vi "Find Cell.vi"(8 "error in":errorcluster, 9 "Lexical Index":string, 10 "Row":refnum<k24>) -> (0 "error out":errorcluster, 2 "Cell":refnum<k24>)   [LabVIEW 2021, in "Open Xml.lvlib"]
uses:
  Open Xml.lvlib
  D:/git/Open-Xml-LabVIEW/Source/DocumentFormat.OpenXml.dll
  DocumentFormat.OpenXml.dll
  D:/git/Open-Xml-LabVIEW/Source/DocumentFormat.OpenXml.Framework.dll
  DocumentFormat.OpenXml.Framework.dll
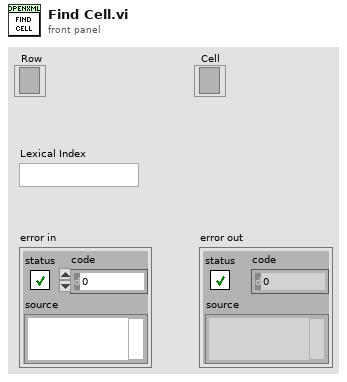
[diagram p1: front panel]
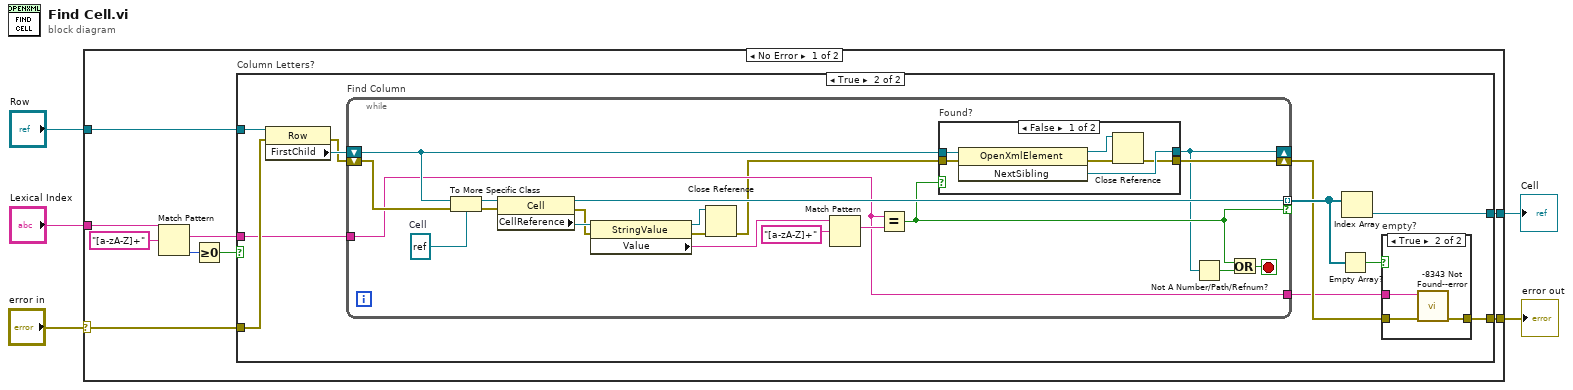
[diagram p0: block diagram]
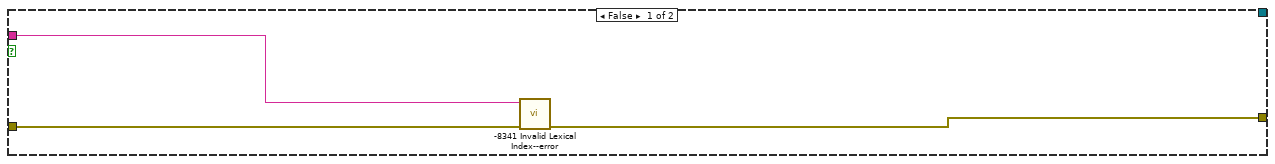
[diagram p2: hidden frame]
diagram:
  n1 = case shown="No Error" "error in" {
    selector: "error in" -> [w13 w61]
    tunnel: "Row" -> [w14 _]
    tunnel: "Lexical Index" -> [w11 _]
    tunnel: [w8 w61] -> w2
    tunnel: [w7 _] -> w1
    frame No Error {
      n2 = Match Pattern(string=w11, regular expression="[a-zA-Z]+") -> (match substring=w10:string, offset past match=w9:i32)  [unwired: 1 in, 2 out]
      n3 = Greater Or Equal To 0?(x=w9) -> (x >= 0?=w6:bool)
      n4 = case "Column Letters?" shown="True" w6 {
        tunnel: w14 -> [_ w28]
        tunnel: w13 -> [w17 w27]
        tunnel: w10 -> [w15 w24]
        tunnel: [w16 w18] -> w8
        tunnel: [_ w23] -> w7
        frame False {
          n5 = call "-8341 Invalid Lexical Index--error.vi"("error in"=w17, "Lexical Index"=w15) -> ("error out"=w16:errorcluster)  [unwired: 9 in]
        }
        frame True {
          n6 = property class="Row"(reference=w28, error in=w27) -> (error out=w25:errorcluster, "FirstChild"=w26:refnum<k24>)  [unwired: 1 out]
          n7 = while "Find Column" {
            shift-right: [w46] -> w20
            shift-left: w25 -> [w52]
            shift-right: [w37] -> _
            shift-left: w26 -> [w36]
            tunnel: [w48] -> w22 mode=indexing if=w38
            tunnel: w24 -> [w35]
            tunnel: [w35] -> w19
            stop <- w50 stop-if-true
            w45 = refnum<k24> refnum  # Cell
            n8 = To More Specific Class(target class=w45, reference=w36, error in=w52) -> (specific class reference=w49:refnum<k24>, error out=w47:errorcluster)
            n9 = property class="Cell"(reference=w49, error in=w47) -> (reference out=w48:refnum<k24>, error out=w42:errorcluster, "CellReference"=w44:refnum<k24>)
            n10 = property class="StringValue"(reference=w44, error in=w42) -> (reference out=w33:refnum<k24>, error out=w43:errorcluster, "Value"=w40:string)
            n11 = Close Reference(reference=w33, error in (no error)=w43) -> (error out=w34:errorcluster)
            n12 = Match Pattern(string=w40, regular expression="[a-zA-Z]+") -> (match substring=w39:string)  [unwired: 1 in, 3 out]
            n13 = Equal?(x=w35, y=w39) -> (x = y?=w38:bool)
            n14 = case "Found?" shown="False" w38 {
              tunnel: [w54 w59] -> w46
              tunnel: w36 -> [w57 w60]
              tunnel: [w55 w60] -> w37
              tunnel: w34 -> [w56 w59]
              frame False {
                n15 = invoke class="OpenXmlElement" method="NextSibling"(reference=w57, error in=w56) -> (reference out=w53:refnum<k24>, error out=w58:errorcluster, "NextSibling"=w55:refnum<k24>)  [unwired: 1 in]
                n16 = Close Reference(reference=w53, error in (no error)=w58) -> (error out=w54:errorcluster)
              }
              frame True {
              }
            }
            n17 = Not A Number/Path/Refnum?(number/path/refnum=w37) -> (NaN/Path/Refnum?=w51:bool)
            n18 = Or(x=w38, y=w51) -> (x .or. y?=w50:bool)
          }
          n19 = Empty Array?(array=w22) -> (empty?=w21:bool)
          n20 = Index Array(array=w22) -> (element=w23:refnum<k24>)  [unwired: 1 in]
          n21 = case "empty?" shown="True" w21 {
            tunnel: w20 -> [w29 w32]
            tunnel: w19 -> [_ w31]
            tunnel: [w29 w30] -> w18
            frame False {
            }
            frame True {
              n22 = call "-8343 Not Found--error.vi"("error in (no error)"=w32, "Item"=w31) -> ("error out"=w30:errorcluster)  [unwired: 9 in]
            }
          }
        }
      }
    }
    frame Error {
    }
  }
  "error out" <- w2
  "Cell" <- w1
